vi "脉冲宽度测量.vi"() -> ()   [LabVIEW 2010]
doc: "I. Description:\nThis example demonstrates how to measure pulse width on a Counter Input Channel. The Starting Edge, Minimum Value and Maximum Value are all configurable. \n\nThis example shows how to measure pulse width on the counter's default input terminal (refer to section IV, I/O Connections Overview, below for more information), but could easily be expanded to measure pulse width on any PFI, RTSI, or internal signal.\n\nII. Instructions for Running:\n1. Select the Physical Channel which corresponds to the counter you want to measure pulse width on the DAQ device.\n2. Enter the measurement Edge to specify what type of pulse you want the counter to measure. Enter the Maximum and Minimum Value to specify the range or your unknown pulse width. Additionally, you can change the input terminal where the pulse width is measured using the channel property node.\nNote: It is important to set the Maximum and Minimum Values of your unknown pulse as accurately as possible so the best internal timebase can be chosen to minimize measurement error. The default values specify a range that can be measured by the counter using the 20MhzTimebase. Use the Gen Dig Pulse example to verify that you are measuring correctly on the DAQ device.\n\nIII. Block Diagram Steps:\n1. Create a Counter Input channel to measure Pulse Width. The Edge parameter is used to determine if the counter will measure high or low pulses. It is important to set the Maximum and Minimum Values of your unknown pulse as accurately as possible so the best internal timebase can be chosen to minimize measurement error. The default values specify a range that can be measured by the counter using the 20MhzTimebase.\n2. Call the Read VI to return the next pulse width measurement. Set a timeout so an error is returned if a pulse is not returned in the specified time limit.\n3. Call the Clear Task VI to clear the Task \n4. Use the popup dialog box to display an error if any.\n\nIV. I/O Connections Overview:\nThe counter will measure pulses on the input terminal of the counter specified in the Physical Channel I/O control. \n\nIn this example the pulse width will be measured on the default input terminal on ctr0. \n\nFor more information on the default counter input and output terminals for your device, open the NI-DAQmx Help, and refer to Counter Signal Connections found under the Device Considerations book in the table of contents."
uses:
  <vilib>/Utility/error.llb/DialogType.ctl
  <vilib>/DAQmx/read.llb/DAQmx Read (Counter DBL 1Chan 1Samp).vi
  <vilib>/DAQmx/create/channels.llb/DAQmx Create Channel (CI-Pulse Width).vi
  <vilib>/daqmx/miscellaneous.llb/DAQmx Fill In Error Info.vi
panel:
  out "Measured Pulse Width (sec)":dbl format="%0.9f"
  # "For instructions, select Help>>Show Context Help"
  # "Channel Parameters"
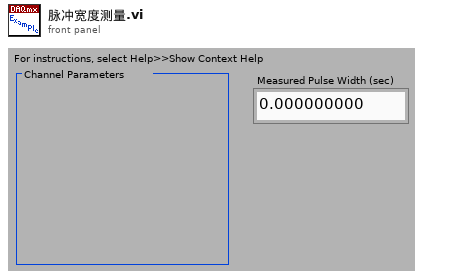
[diagram p1: front panel]
types:
  T1 = typedef "DialogType.ctl" = u16
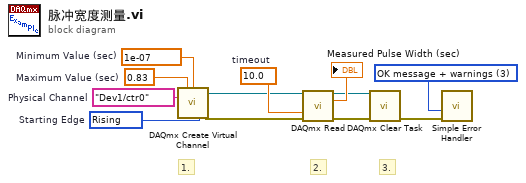
[diagram p0: block diagram]
diagram:
  w5 = 10280 items=["Rising"=10280, "Falling"=10171]  # Starting Edge
  w10 = tag "Dev1/ctr0"  # Physical Channel
  w11 = 0.83  # Maximum Value (sec)
  w12 = 1e-07  # Minimum Value (sec)
  w4 = T1 3 items=["no dialog", "OK message", "continue or stop message", "OK message + warnings", "continue/stop + warnings"] ("type of dialog (OK msg:1)")
  w9 = 10.0  # timeout
  # "3."
  # "2."
  # "1."
  n1 = call-poly <vilib>:"DAQmx Create Virtual Channel.vi"("maximum value"=w11, "minimum value"=w12, "counter"=w10, "starting edge"=w5) -> ("task out"=w8:refnum<k21>, "error out"=w7:errorcluster)  [unwired: 10 in]
  n2 = call-poly <vilib>:"DAQmx Read.vi"("task/channels in"=w8, "timeout"=w9, "error in"=w7) -> ("task out"=w3:refnum<k21>, "data"=→"Measured Pulse Width (sec)":dbl, "error out"=w2:errorcluster)  [unwired: 10 in]
  n3 = call <vilib>:"DAQmx Clear Task.vi"("task in"=w3, "error in"=w2) -> ("error out"=w1:errorcluster)  [unwired: 13 in]
  n4 = call <vilib>:"Simple Error Handler.vi"("type of dialog (OK msg:1)"=w4, "error in (no error)"=w1) -> ()  [unwired: 3 in, 5 out]
